vi "Property Node_Selected Element.vi"(7 "Action":T1, 8 "error in (no error)":errorcluster, 11 "Affected Items":T2) -> (0 "error out":errorcluster, 1 "Selected Property Label":string, 2 "index of element":i32, 3 "Selected Element Term Refnum":refnum<vi>, 4 "Display String":string, 6 "Element details":cluster{"First":bool, "Last":bool})   [LabVIEW 2023]
doc: "Get index of clicked element in property node, the name of the node and whether it's first or last in the node (element details)."
uses:
  top/BundleMagic.ctl
  controls/action enum.ctl
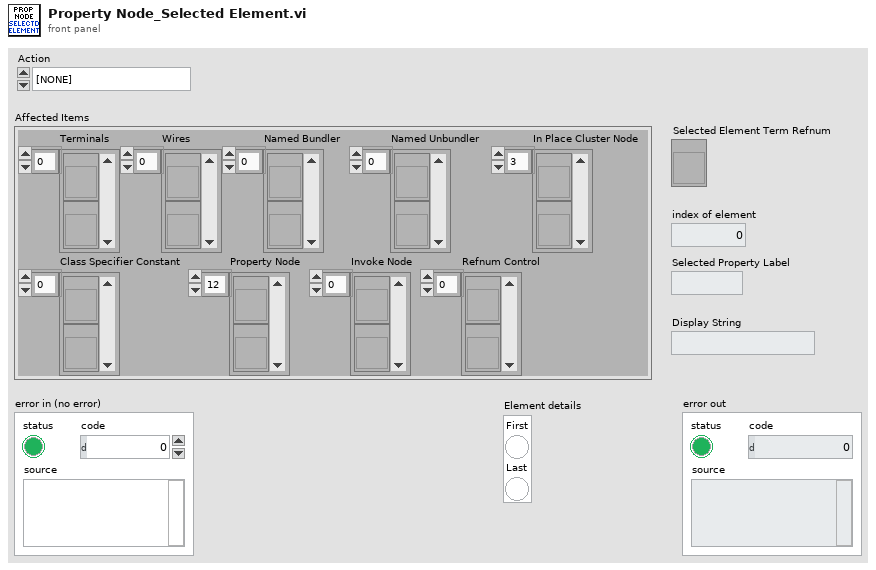
[diagram p1: front panel]
types:
  T1 = typedef "action enum.ctl" = enum16{"[NONE]", "Wire Bundle", "Wire Unbundle", "Terminal Unbundle", "Terminal Bundle", "Bundler Move Up", "Bundler Move Down", "Bundler Insert", "Bundler Remove", "Bundler Remove Unwired", "Bundler Rearrange", "In Place Insert", "In Place Remove", "In Place Remove Unwired", "In Place Rearrange", "Wire Properties", "Wire Method", "Terminal Properties", "Terminal Method", "Property Move Up", "Property Move Down", "Properties Insert", "Properties Remove", "Properties Remove Unwired", "Properties Rearrange", "Method Change", "Class for Constant", "Class For Control", "Class For Node", "Class Name to Clipboard"}
  T2 = typedef "BundleMagic.ctl" = cluster{"Terminals":refnum<vi>[], "Wires":refnum<vi>[], "Named Bundler":refnum<vi>[], "Named Unbundler":refnum<vi>[], "In Place Cluster Node":refnum<vi>[], "Class Specifier Constant":refnum<vi>[], "Property Node":refnum<vi>[], "Invoke Node":refnum<vi>[], "Refnum Control":refnum<vi>[]}
  T3 = enum16{"[NONE]", "Wire Bundle", "Wire Unbundle", "Terminal Unbundle", "Terminal Bundle", "Bundler Insert", "Bundler Remove", "Bundler Remove Unwired", "Bundler Rearrange", "In Place Insert", "In Place Remove", "In Place Remove Unwired", "In Place Rearrange", "Wire Properties", "Wire Method", "Terminal Properties", "Terminal Method", "Properties Insert", "Properties Remove", "Properties Remove Unwired", "Properties Rearrange", "Method Change", "Class for Constant", "Class For Control", "Class For Node", "Class Name to Clipboard"}
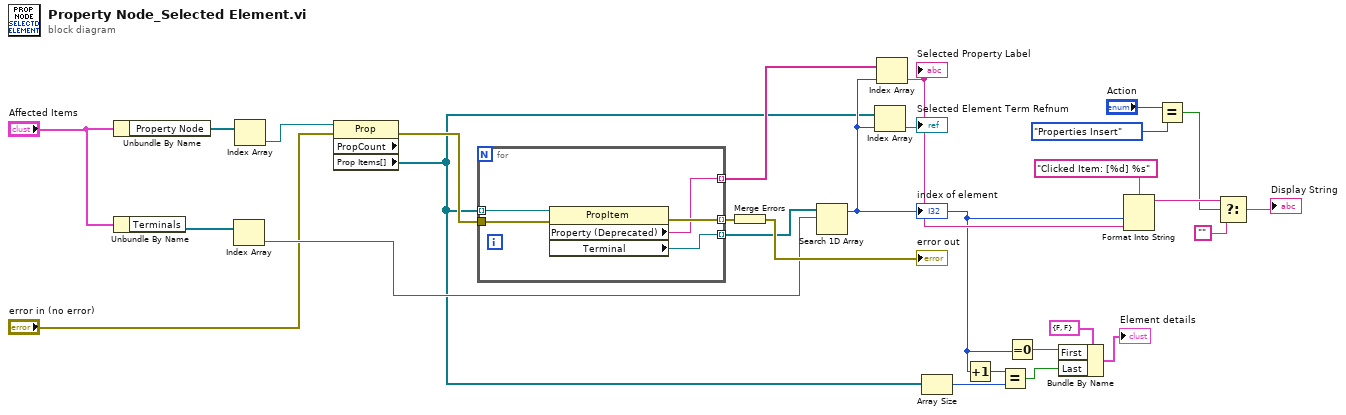
[diagram p0: block diagram]
diagram:
  n1 = Unbundle By Name("Affected Items") -> ("Property Node"=w21:refnum<vi>[])
  n2 = Unbundle By Name("Affected Items") -> ("Terminals"=w20:refnum<vi>[])
  n3 = Index Array(array=w20) -> (element=w23:refnum<vi>)  [unwired: 1 in]
  n4 = Index Array(array=w21) -> (element=w28:refnum<vi>)  [unwired: 1 in]
  n5 = property class="Prop" props=["PropCount", "Prop Items[]"](reference=w28, error in="error in (no error)") -> (error out=w24:errorcluster, "Prop Items[]"=w3:refnum<vi>[])  [unwired: 2 out]
  n6 = for {
    tunnel: w3 -> [w33] mode=indexing
    tunnel: [w31] -> w22 mode=indexing
    tunnel: w24 -> [w32]
    tunnel: [w30] -> w25 mode=indexing
    tunnel: [w29] -> w17 mode=indexing
    n7 = property class="PropItem"(reference=w33, error in=w32) -> (error out=w30:errorcluster, "Property (Deprecated)"=w29:string, "Terminal"=w31:refnum<vi>)  [unwired: 1 out]
  }
  n8 = Merge Errors(w25) -> (→"error out":errorcluster)
  n9 = Search 1D Array(1D array=w22, element=w23) -> (index of element=w5:i32)  [unwired: 1 in]
  "index of element" <- w5
  n10 = Index Array(array=w3, index=w5) -> (element=→"Selected Element Term Refnum":refnum<vi>)
  n11 = Index Array(array=w17, index=w5) -> (element=w15:string)
  "Selected Property Label" <- w15
  n12 = Array Size(array=w3) -> (size(s)=w2:i32)
  n13 = Increment(x=w5) -> (x+1=w4:i32)
  n14 = Equal?(x=w4, y=w2) -> (x = y?=w1:bool)
  n15 = Equal To 0?(x=w5) -> (x = 0?=w6:bool)
  n16 = Bundle By Name(cluster=cluster{"First":bool, "Last":bool} {"First"=FALSE, "Last"=FALSE} ("Element details"), "First"=w6, "Last"=w1) -> (→"Element details":cluster{"First":bool, "Last":bool})
  n17 = Format Into String(format string="Clicked Item: [%d] %s", w5, w15) -> (resulting string=w12:string)  [unwired: 2 in, 1 out]
  n18 = Equal?(x="Action", y=T3."Properties Insert" ("Action")) -> (x = y?=w11:bool)
  n19 = Select(t=w12, s=w11, f="") -> (s? t:f=→"Display String":string)
